vi "ReadSector.vi"(8 "error In":errorcluster, 10 "Sector":u8=1, 11 "VISA resource In":refnum<visa-resource-name>) -> (0 "error out":errorcluster, 2 "Data Out":u8[](array[numeric]), 3 "VISA resource Out":refnum<visa-resource-name>)   [LabVIEW 2009]
uses:
  Packet.ctl
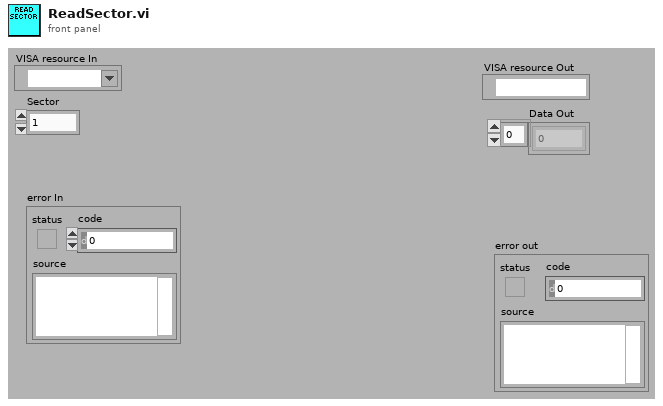
[diagram p1: front panel]
types:
  T1 = typedef "Packet.ctl" = cluster{"Length":u8, "Type":u8, "PID":u8, "Data":u8[], "CRC":u8}
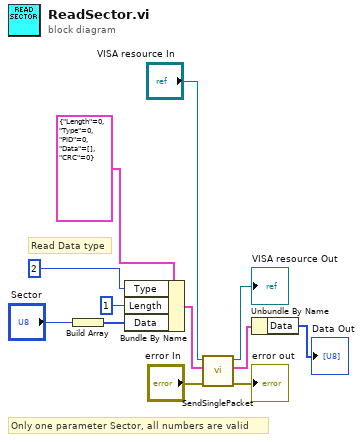
[diagram p0: block diagram]
diagram:
  # "Only one parameter Sector, all numbers are valid"
  # "Read Data type"
  n1 = Build Array("Sector") -> (w9:u8[])
  n2 = Bundle By Name(cluster=T1 {"Length"=0, "Type"=0, "PID"=0, "Data"=[], "CRC"=0} ("Transmit"), "Type"=u8 2, "Length"=u8 1, "Data"=w9) -> (w5:T1)
  n3 = call "SendSinglePacket.vi"("error in (no error)"="error In", "Transmit"=w5, "VISA resource name"="VISA resource In") -> ("error out"=→"error out":errorcluster, "element"=w1:T1, "VISA resource name out"=→"VISA resource Out":refnum<visa-resource-name>)  [unwired: 6 in]
  n4 = Unbundle By Name(w1) -> ("Data"=→"Data Out":u8[])
